vi "Get Mode.vi"(0 "reference in":refnum<class "Simulated-PowerModule.lvclass">, 11 "Error In":errorcluster) -> (4 "reference out":refnum<class "Simulated-PowerModule.lvclass">, 6 "Mode":string, 15 "Error Out":errorcluster)   [LabVIEW 2023, in "Simulated-PowerModule.lvlib" / "Simulated-PowerModule.lvclass"]
uses:
  Simulated-PowerModule.lvclass
  Simulated-PowerModule.lvclass/Simulated-PowerModule.ctl
  Mode.ctl
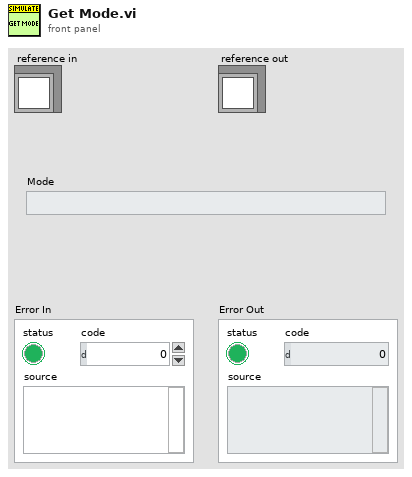
[diagram p1: front panel]
types:
  T1 = typedef "Simulated-PowerModule.lvlib/Simulated-PowerModule.lvclass/Mode.ctl" = u16
  T2 = typedef "Simulated-PowerModule.lvlib/Simulated-PowerModule.lvclass/ObjectAttributes.ctl" = cluster{"JSON Config Path":path, "Configuration":T3, "connected":bool, "reserved":bool, "energized":bool, "output enabled":bool, "setpoint":cluster{"voltage":sgl, "current":sgl, "resistance":sgl}, "last timestamp":i64, "mode":T1, "range":T4, "measurement array":T5[]}
  T3 = typedef "Simulated-PowerModule.lvlib/Simulated-PowerModule.lvclass/Configuration.ctl" = cluster{"range":T4}
  T4 = typedef "PowerModuleInterface.lvlibp/PowerModuleInterface.lvclass/Range.ctl" = cluster{"Current Max (A)":dbl, "Current Min (A)":dbl, "Voltage Max (V)":dbl, "Voltage Min (V)":dbl}
  T5 = typedef "PowerModuleInterface.lvlibp/PowerModuleInterface.lvclass/Measurements.ctl" = cluster{"measured voltage (V)":dbl, "measured current (A)":dbl, "setpoint voltage (V)":dbl, "setpoint current (A)":dbl, "timestamp":dbl}
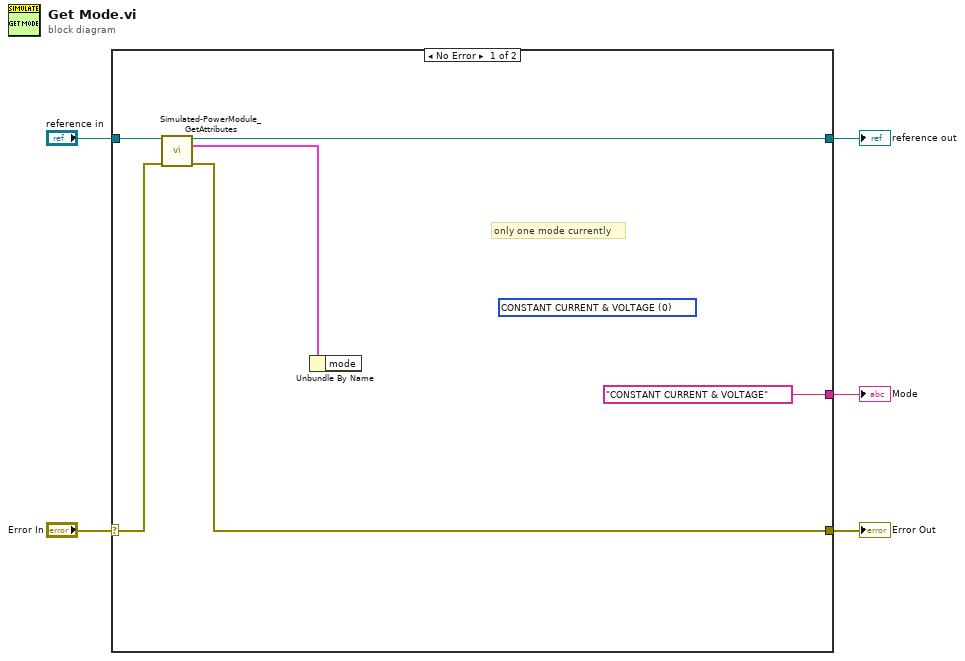
[diagram p0: block diagram]
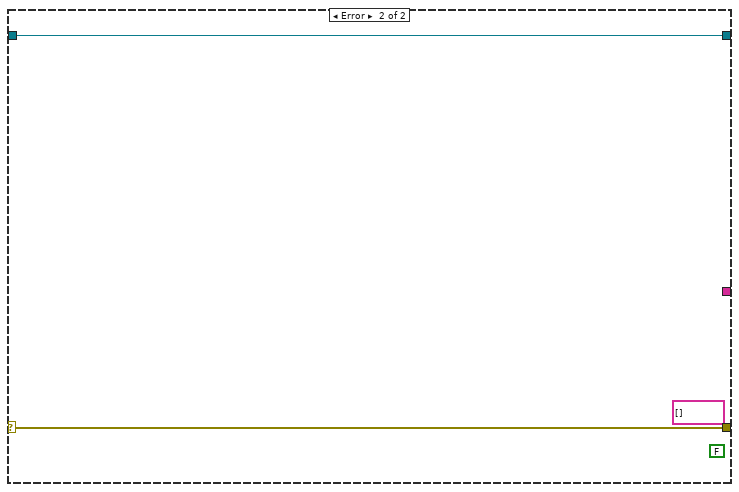
[diagram p2: hidden frame]
diagram:
  n1 = case shown="No Error" "Error In" {
    selector: "Error In" -> [w10 w12]
    tunnel: "reference in" -> [w11 w13]
    tunnel: [w9 w13] -> w2
    tunnel: [w7 w12] -> w3
    tunnel: ["CONSTANT CURRENT & VOLTAGE" ("Mode") _] -> w1
    frame No Error {
      (unwired) T1 0 items=["CONSTANT CURRENT & VOLTAGE"] ("mode")
      # "only one mode currently"
      n2 = call "Simulated-PowerModule_GetAttributes.vi"("reference in"=w11, "Error In"=w10) -> ("reference out"=w9:refnum<class "Simulated-PowerModule.lvclass">, "Data"=w8:T2, "Error Out"=w7:errorcluster)  [unwired: 10 in, 1 out]
      n3 = Unbundle By Name(w8) -> ()  [unwired: 1 out]
    }
    frame Error {
      (unwired) string[] []
      (unwired) FALSE
    }
  }
  "Error Out" <- w3
  "reference out" <- w2
  "Mode" <- w1
